vi "Test Function 3.vi"(1 "x":refnum<class "Dual.lvclass">) -> (0 "f(x)":refnum<class "Dual.lvclass">)   [LabVIEW 2020, in "Tests.lvlib"]
uses:
  Tests.lvlib
  classes/Dual/Dual.lvclass
  classes/Dual/Dual.lvclass/Dual.ctl
  ea8a822e-19c0-451d-95fd-cb421ab043da.vi
  c738264e-79a7-4ccc-b5b2-8c64c8abb521.vi
  ea8a822e-19c0-451d-95fd-cb421ab043da.vi/957074e8-cc3b-4647-8ff1-d975a744cd4e.vi
  classes/Dual/Write a and b.vi
  classes/Dual/Read a and b.vi
  c738264e-79a7-4ccc-b5b2-8c64c8abb521.vi/dd5be0c0-ba72-46c3-966c-165139a40946.vi
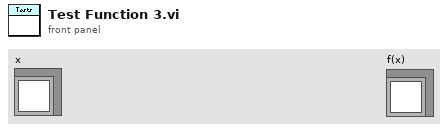
[diagram p1: front panel]
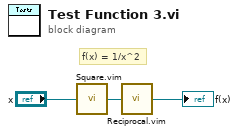
[diagram p0: block diagram]
diagram:
  # "f(x) = 1/x^2"
  n1 = call "Square.vim"("x"="x") -> ("x^2"=w1:refnum<class "Dual.lvclass">)
  n2 = call "Reciprocal.vim"("x"=w1) -> ("1/x"=→"f(x)":refnum<class "Dual.lvclass">)
